vi "edittest handle new sequence.vi"(6 "User Information":T2, 8 "error in (no error)":errorcluster, 10 "New Name Suggestion\n(empty - \"Username Sequence N\")":string, 11 "Connection Refnum":T3) -> (0 "error out":errorcluster, 1 "First Matching Sequence Record":T1, 2 "New Sequence Record":T1, 3 "Connection Refnum":T3, 4 "Existed?":bool)   [LabVIEW 2011]
uses:
  server/database/Sequences/Sequence Record.ctl
  SI.LIB/ODBC/SQL Controls/Connection Refnum.ctl
  server/database/Users/User Record.ctl
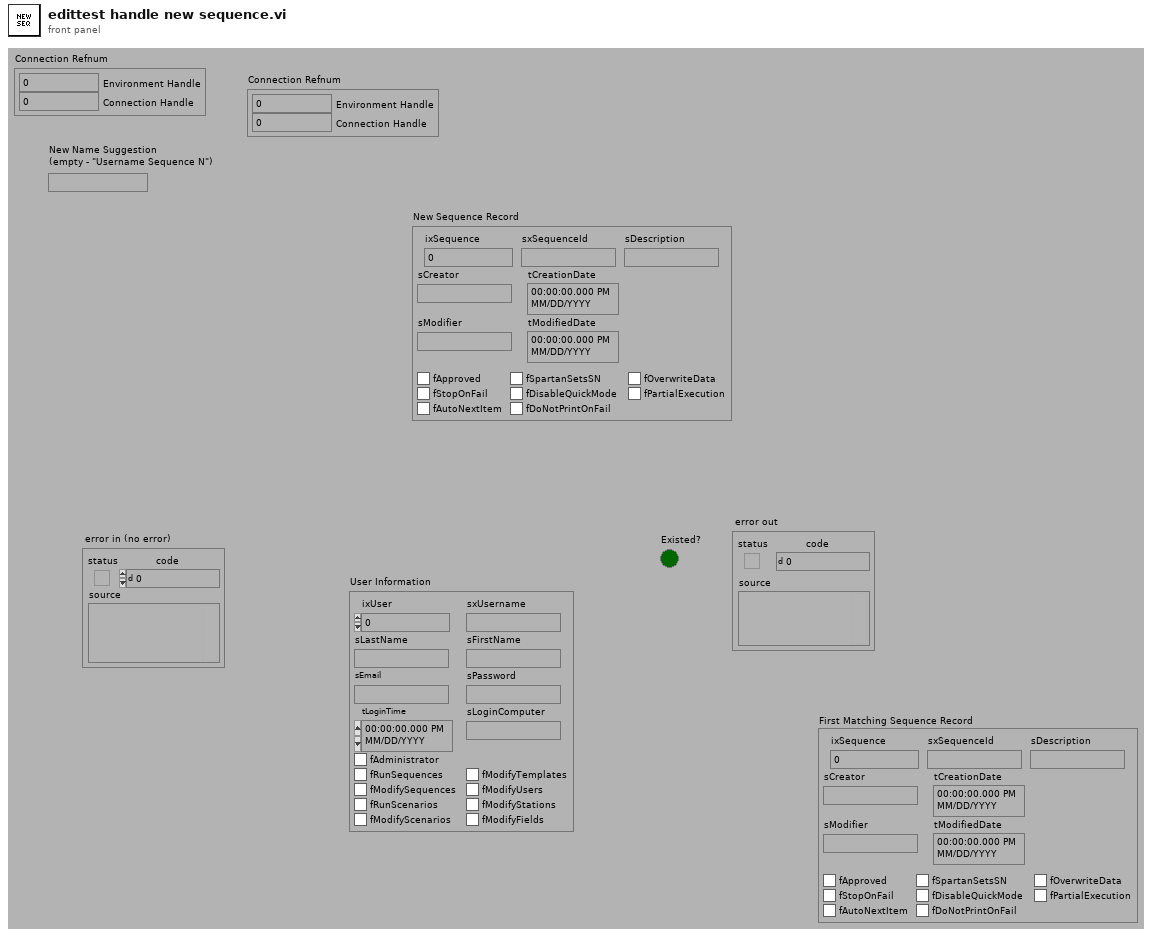
[diagram p1: front panel]
types:
  T1 = typedef "Sequence Record.ctl" = cluster{"ixSequence":i32, "sxSequenceId":string, "sDescription":string, "sCreator":string, "tCreationDate":timestamp, "sModifier":string, "tModifiedDate":timestamp, "fApproved":bool, "fSpartanSetsSN":bool, "fOverwriteData":bool, "fStopOnFail":bool, "fDisableQuickMode":bool, "fPartialExecution":bool, "fAutoNextItem":bool, "fDoNotPrintOnFail":bool}
  T2 = typedef "User Record.ctl" = cluster{"ixUser":i32, "sxUsername":string, "sLastName":string, "sFirstName":string, "sEmail":string, "sPassword":string, "tLoginTime":timestamp, "sLoginComputer":string, "fAdministrator":bool, "fRunSequences":bool, "fModifySequences":bool, "fRunScenarios":bool, "fModifyScenarios":bool, "fModifyTemplates":bool, "fModifyUsers":bool, "fModifyStations":bool, "fModifyFields":bool}
  T3 = typedef "Connection Refnum.ctl" = cluster{"Environment Handle":i32, "Connection Handle":i32}
  T4 = typedef "Keyed Array.ctl" = cluster{"keys":string[], "values":string[]}
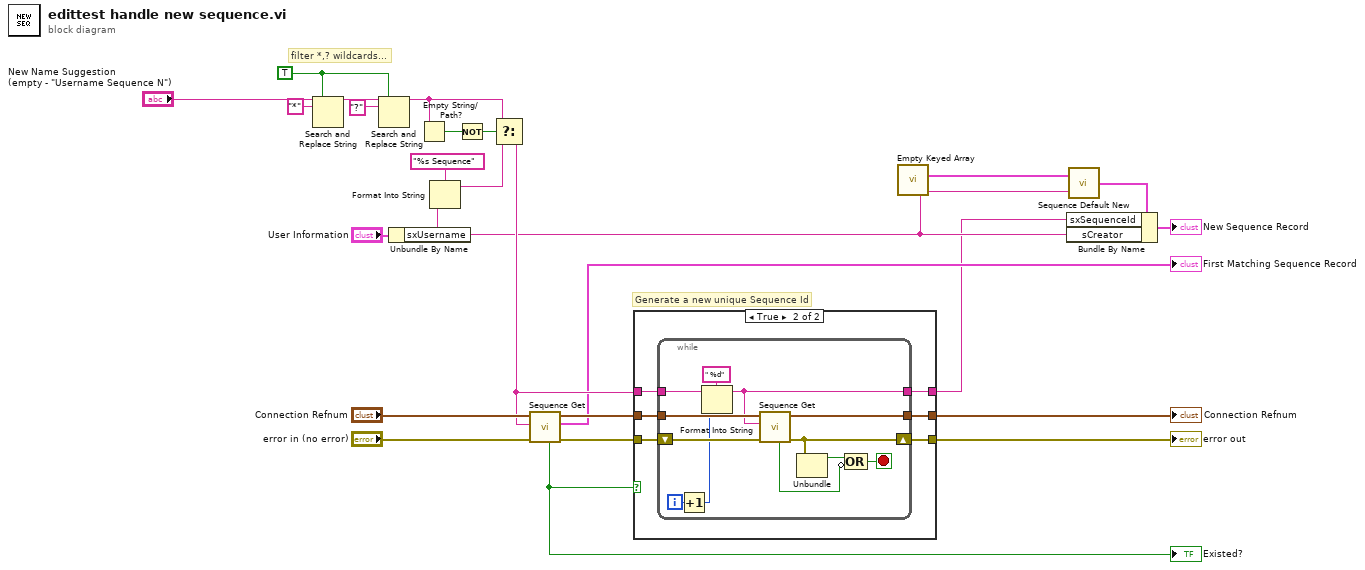
[diagram p0: block diagram]
diagram:
  w4 = TRUE ("replace all? (F)")
  # "filter *,? wildcards..."
  # "Generate a new unique Sequence Id"
  n1 = Search and Replace String(replace all?=w4, input string="New Name Suggestion\n(empty - \"Username Sequence N\")", search string="*") -> (result string=w5:string)  [unwired: 1 in, 7 out]
  n2 = Search and Replace String(replace all?=w4, input string=w5, search string="?") -> (result string=w1:string)  [unwired: 1 in, 7 out]
  n3 = Unbundle By Name("User Information") -> ("sxUsername"=w10:string)
  n4 = Empty String/Path?(string/path=w1) -> (empty?=w22:bool)
  n5 = Format Into String(format string="%s Sequence", w10) -> (resulting string=w20:string)  [unwired: 2 in, 1 out]
  n6 = Not(x=w22) -> (.not. x?=w21:bool)
  n7 = Select(t=w1, s=w21, f=w20) -> (s? t:f=w14:string)
  n8 = call "Sequence Get.vi"("error in (no error)"="error in (no error)", "sxSequenceId (\"\")"=w14, "Connection Refnum"="Connection Refnum") -> ("error out"=w15:errorcluster, "Sequence Record"=→"First Matching Sequence Record":T1, "Connection Refnum"=w17:T3, "Data Present"=w8:bool)  [unwired: 5 out]
  "Existed?" <- w8
  n9 = case shown="True" w8 {
    tunnel: [w27 w34] -> w19
    tunnel: [w28 w33] -> w7
    tunnel: w17 -> [w27 w32]
    tunnel: w15 -> [w26 w31]
    tunnel: w14 -> [w28 w30]
    tunnel: [w26 w29] -> w13
    frame False {
    }
    frame True {
      n10 = while {
        shift-right: [w40] -> w29
        shift-left: w31 -> [w46]
        tunnel: w30 -> [w43]
        tunnel: w32 -> [w45]
        tunnel: [w39] -> w34
        tunnel: [w37] -> w33
        i -> [w36]
        stop <- w41 stop-if-true
        n11 = Increment(x=w36) -> (x+1=w35:i32)
        n12 = Format Into String(format string=" %d", initial string=w43, w35) -> (resulting string=w37:string)  [unwired: 1 in, 1 out]
        n13 = call "Sequence Get.vi"("error in (no error)"=w46, "sxSequenceId (\"\")"=w37, "Connection Refnum"=w45) -> ("error out"=w40:errorcluster, "Connection Refnum"=w39:T3, "Data Present"=w38:bool)  [unwired: 6 out]
        n14 = Unbundle(w40) -> ("status"=w42:bool)  [unwired: 2 out]
        n15 = Compound Arithmetic op=OR(w42, invert w38) -> (w41:bool)
      }
    }
  }
  "error out" <- w13
  "Connection Refnum" <- w19
  n16 = call "Empty Keyed Array.vi"() -> ("empty keyed array"=w12:T4)  [unwired: 3 out]
  n17 = call "Sequence Default New.vi"("Username"=w10, "Post Data"=w12) -> ("Default New Instrument"=w25:T1)
  n18 = Bundle By Name(cluster=w25, "sxSequenceId"=w7, "sCreator"=w10) -> (→"New Sequence Record":T1)
